vi "CalculatedotProduct.vi"(8 "qb (in)":T1, 11 "qa (in)":T1) -> (3 "Quat Product":dbl)   [LabVIEW 2015]
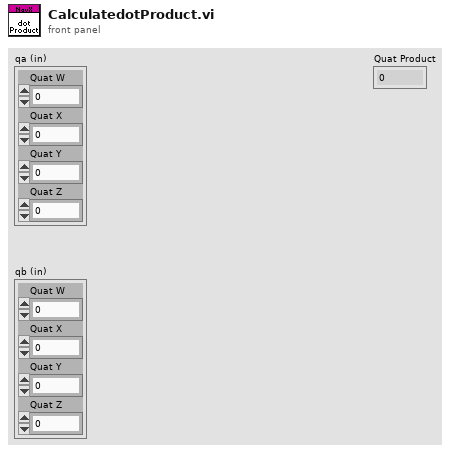
[diagram p1: front panel]
types:
  T1 = cluster{"Quat W":dbl, "Quat X":dbl, "Quat Y":dbl, "Quat Z":dbl}
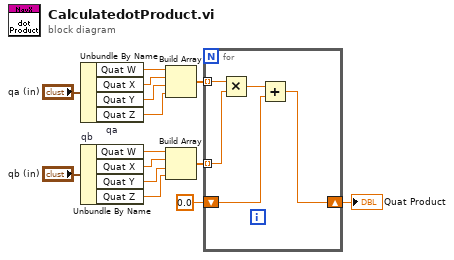
[diagram p0: block diagram]
diagram:
  n1 = Unbundle By Name "qa"("qa (in)") -> ("Quat W"=w5:dbl, "Quat X"=w6:dbl, "Quat Y"=w7:dbl, "Quat Z"=w8:dbl)
  n2 = Unbundle By Name "qb"("qb (in)") -> ("Quat W"=w9:dbl, "Quat X"=w10:dbl, "Quat Y"=w11:dbl, "Quat Z"=w12:dbl)
  n3 = Build Array(w5, w6, w7, w8) -> (w13:dbl[])
  n4 = Build Array(w9, w10, w11, w12) -> (w14:dbl[])
  n5 = for {
    tunnel: w13 -> [w19] mode=indexing
    tunnel: w14 -> [w17] mode=indexing
    shift-right: [w15] -> w1
    shift-left: 0.0 -> [w16]
    n6 = Multiply(x=w19, y=w17) -> (x*y=w18:dbl)
    n7 = Add(x=w18, y=w16) -> (x+y=w15:dbl)
  }
  "Quat Product" <- w1
